vi "set freq correction.vi"(8 "error in (no error)":errorcluster, 10 "Frequency Correction (ppm)":i32, 11 "DeviceRefnum":u64) -> (0 "error out":errorcluster, 2 "function return":i32, 3 "DeviceRefnum Out":u64)   [LabVIEW 2015, in "rtlsdr.lvlib"]
doc: "Set the frequency correction value for the device."
uses:
  rtlsdr.lvlib
  rtlsdr/rtlsdr.dll
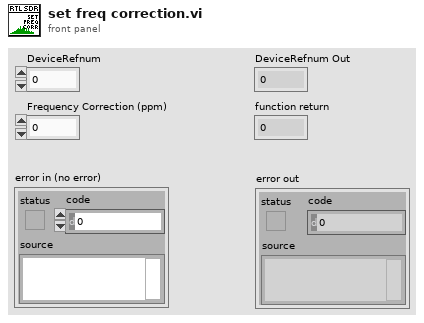
[diagram p1: front panel]
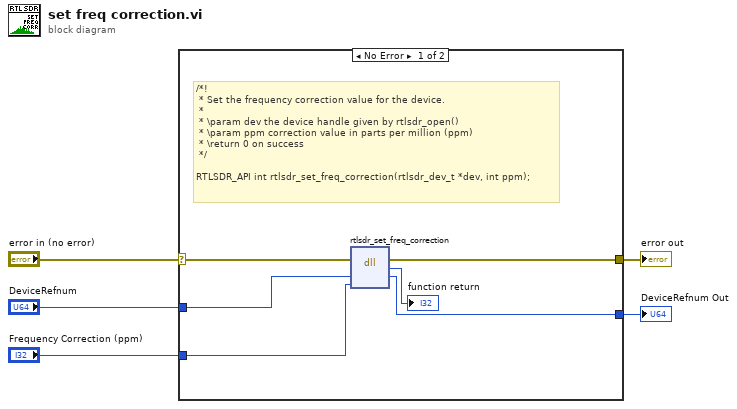
[diagram p0: block diagram]
diagram:
  n1 = case shown="No Error" "error in (no error)" {
    selector: "error in (no error)" -> [w6 w12]
    tunnel: [w10 w12] -> w5
    tunnel: "DeviceRefnum" -> [w9 w13]
    tunnel: "Frequency Correction (ppm)" -> [w8 _]
    tunnel: [w7 w13] -> w2
    frame No Error {
      # "/*!\n * Set the frequency correction value for the device.\n *\n * \\param dev the device handle given by rtlsdr_open()\n * \\param ppm correction value in parts per million (ppm)\n * \\return 0 on success\n */\n\nRTLSDR_API int rtlsdr_set_freq_correction(rtlsdr_dev_t *dev, int ppm);"
      n2 = dll-call lib="C:/Users/TheDoctor/Documents/Projects/Labview Libraries/rtlsdr/rtlsdr.*" fn="rtlsdr_set_freq_correction"(error in=w6, "DeviceRefnum"=w9, "Frequency Correction (ppm)"=w8) -> (error out=w10:errorcluster, "return type"=→"function return":i32, "DeviceRefnum"=w7:u64)  [unwired: 3 in, 1 out]
    }
    frame Error {
    }
  }
  "error out" <- w5
  "DeviceRefnum Out" <- w2
